vi "Modify Tank.vi"(0 "Original":T1[](array[typedef]), 5 "wheelbase_width":dbl, 11 "error in":errorcluster) -> (4 "original":T1[](array[typedef]), 6 "left":T1[](array[typedef]), 8 "right":T1[](array[typedef]), 15 "error out":errorcluster)   [LabVIEW 2017, in "Pathfinder.lvlib"]
doc: "CAPI void pathfinder_modify_tank(Segment *original, int length, Segment *left, Segment *right, double wheelbase_width);"
uses:
  Pathfinder.lvlib
  Segment.ctl
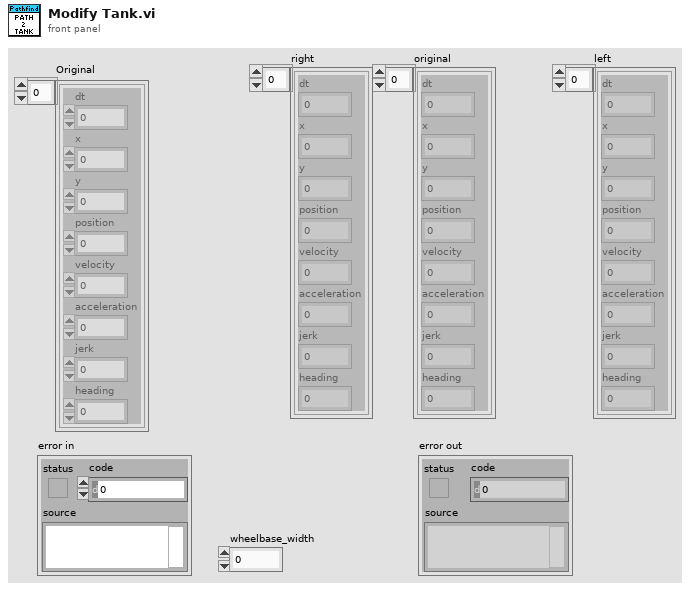
[diagram p1: front panel]
types:
  T1 = typedef "Pathfinder.lvlib/Segment.ctl" = cluster{"dt":dbl, "x":dbl, "y":dbl, "position":dbl, "velocity":dbl, "acceleration":dbl, "jerk":dbl, "heading":dbl}
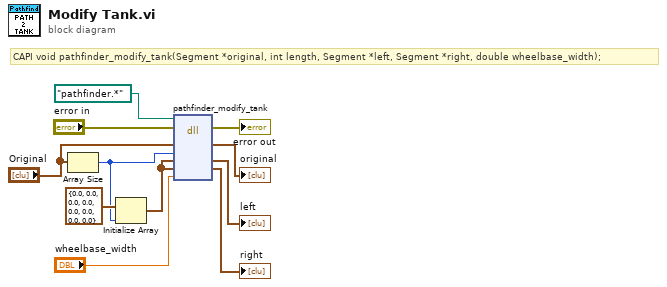
[diagram p0: block diagram]
diagram:
  # "CAPI void pathfinder_modify_tank(Segment *original, int length, Segment *left, Segment *right, double wheelbase_width);"
  n1 = Array Size(array="Original") -> (size(s)=w5:i32)
  n2 = Initialize Array(T1 {"dt"=0.0, "x"=0.0, "y"=0.0, "position"=0.0, "velocity"=0.0, "acceleration"=0.0, "jerk"=0.0, "heading"=0.0} ("segment"), w5) -> (w7:T1[])
  n3 = dll-call lib="?" fn="pathfinder_modify_tank"(path in=path "pathfinder.*", error in="error in", "original"="Original", "length"=w5, "left"=w7, "right"=w7, "wheelbase_width"="wheelbase_width") -> (error out=→"error out":errorcluster, "original"=→"original":T1[], "left"=→"left":T1[], "right"=→"right":T1[])  [unwired: 4 in, 1 out]
